vi "Disconnect.vi"(8 "error in (no error)":errorcluster, 11 "TC01 in":refnum<class "TC01K.lvclass">) -> (0 "error out":errorcluster, 3 "TC01 out":refnum<class "TC01K.lvclass">)   [LabVIEW 2018, in "TC01K.lvlib" / "TC01K.lvclass"]
uses:
  TC01K.lvclass
  builds/Thermocouple.lvlibp/Thermocouple.lvclass
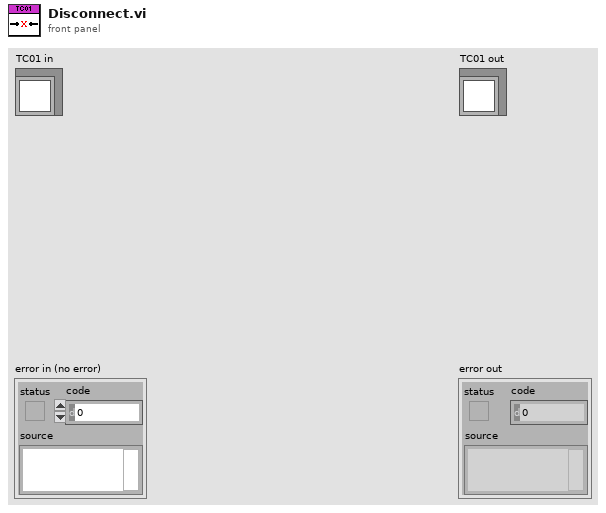
[diagram p1: front panel]
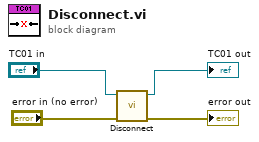
[diagram p0: block diagram]
diagram:
  n1 = call-parent "Disconnect.vi"("error in (no error)"="error in (no error)", "Thermocouple in"="TC01 in") -> ("error out"=→"error out":errorcluster, "Thermocouple out"=→"TC01 out":refnum<class "TC01K.lvclass">)  [unwired: 8 in]
